vi "Update UI.vi"(8 "error in (no error)":errorcluster, 11 "Call Actor in":refnum<class "Call Actor.lvclass">) -> (0 "error out":errorcluster, 3 "Call Actor out":refnum<class "Call Actor.lvclass">)   [LabVIEW 2020, in "Call Actor.lvlib" / "Call Actor.lvclass"]
uses:
  Call Actor.lvclass
  Call Actor.lvclass/Call Actor.ctl
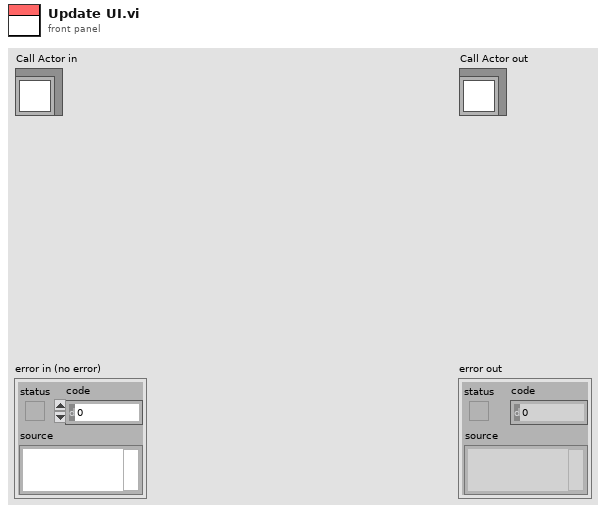
[diagram p1: front panel]
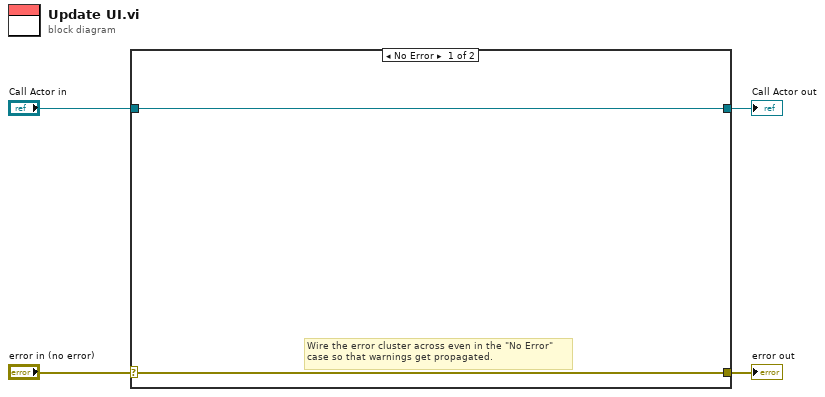
[diagram p0: block diagram]
diagram:
  n1 = case shown="No Error" "error in (no error)" {
    selector: "error in (no error)" -> [w5 w8]
    tunnel: [w5 w8] -> w3
    tunnel: [w6 w7] -> w1
    tunnel: "Call Actor in" -> [w6 w7]
    frame No Error {
      # "Wire the error cluster across even in the \"No Error\"\ncase so that warnings get propagated."
    }
    frame Error {
    }
  }
  "error out" <- w3
  "Call Actor out" <- w1
